vi "FPGA.vi"(7 "LabVIEW Web Service Request":refnum<class "Web Request.lvclass">, 9 "getdata":dbl, 10 "stop":dbl, 11 "save_file":dbl) -> (1 "Chassis Temperature":dbl, 2 "value":string)   [LabVIEW 2020]
uses:
  <vilib>/wsapi/Web Request.lvclass
panel:
  # "Use the Web Service Request input terminal to call the VIs on the Web Services palette. Do not remove it from the connector pane unless you don't need access to the palette."
  # "Each additional control wired to the connector pane will be available as an input in the URL. To include an indicator in terminal-mode output (the default setting), it must also be wired to the connector pane."
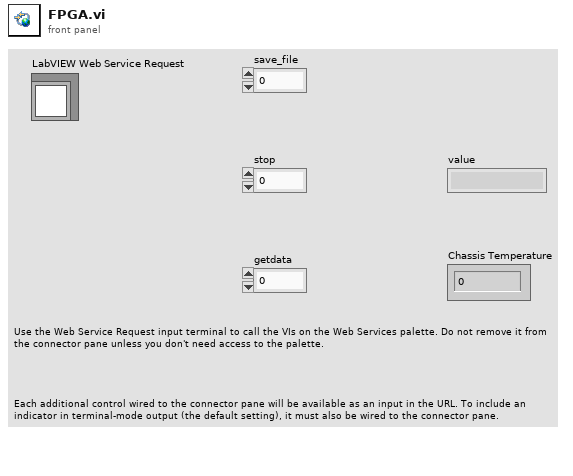
[diagram p1: front panel]
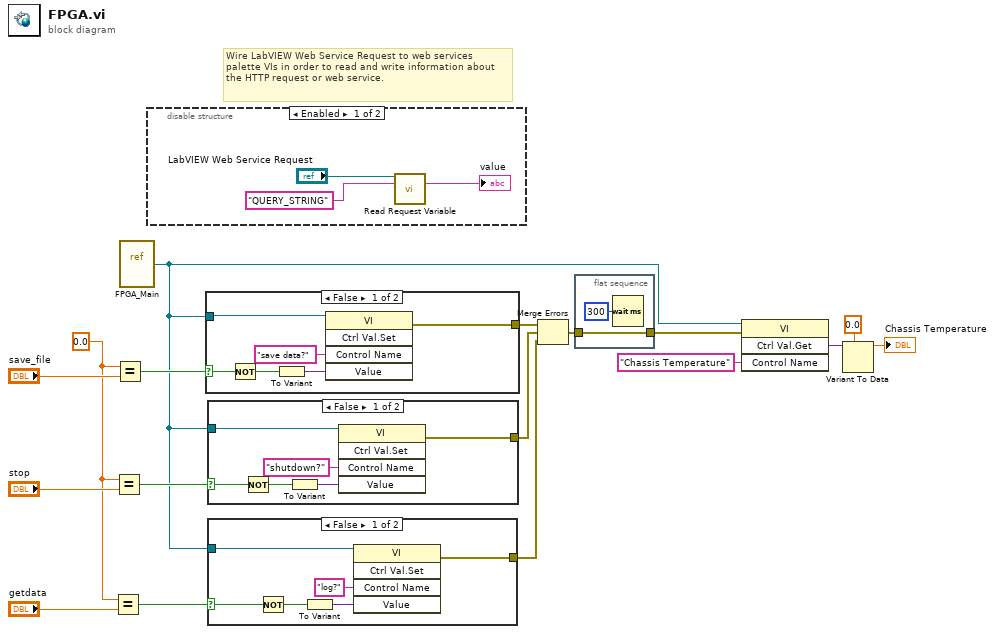
[diagram p0: block diagram]
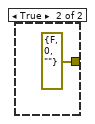
[diagram p2: hidden frame]
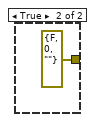
[diagram p3: hidden frame]
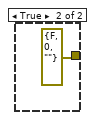
[diagram p4: hidden frame]
diagram:
  w10 = 0.0 ("x")
  # "Wire LabVIEW Web Service Request to web services palette VIs in order to read and write information about the HTTP request or web service."
  n1 = Equal?(x=w10, y="getdata") -> (x = y?=w8:bool)
  n2 = Equal?(x=w10, y="stop") -> (x = y?=w7:bool)
  n3 = Equal?(x=w10, y="save_file") -> (x = y?=w9:bool)
  n4 = vi-ref "FPGA_Main.vi"() -> (w6:refnum<vi>)
  n5 = disable-structure shown="Enabled" {
    frame Enabled {
      n6 = call <vilib>:"Read Request Variable.vi"("LabVIEW Web Service Request"="LabVIEW Web Service Request", "variable name"="QUERY_STRING") -> ("value"=→"value":string)  [unwired: 11 in, 2 out]
    }
    frame Disabled {
    }
  }
  n7 = case shown="False" w9 {
    selector: w9 -> [w25 _]
    tunnel: w6 -> [w26 _]
    tunnel: [w21 errorcluster {"status"=FALSE, "code"=0, "source"=""} ("error out")] -> w3
    frame False {
      n8 = Not(x=w25) -> (.not. x?=w23:bool)
      n9 = To Variant(anything=w23) -> (Variant=w24:variant)
      n10 = invoke class="VI" method="Ctrl Val.Set"(reference=w26, "Control Name"="save data?", "Value"=w24) -> (error out=w21:errorcluster)  [unwired: 2 in, 4 out]
    }
    frame True {
    }
  }
  n11 = case shown="False" w7 {
    selector: w7 -> [w30 _]
    tunnel: w6 -> [w29 _]
    tunnel: [w28 errorcluster {"status"=FALSE, "code"=0, "source"=""} ("error out")] -> w4
    frame False {
      n12 = Not(x=w30) -> (.not. x?=w32:bool)
      n13 = To Variant(anything=w32) -> (Variant=w31:variant)
      n14 = invoke class="VI" method="Ctrl Val.Set"(reference=w29, "Control Name"="shutdown?", "Value"=w31) -> (error out=w28:errorcluster)  [unwired: 2 in, 4 out]
    }
    frame True {
    }
  }
  n15 = case shown="False" w8 {
    selector: w8 -> [w37 _]
    tunnel: w6 -> [w36 _]
    tunnel: [w35 errorcluster {"status"=FALSE, "code"=0, "source"=""} ("error out")] -> w5
    frame False {
      n16 = Not(x=w37) -> (.not. x?=w39:bool)
      n17 = To Variant(anything=w39) -> (Variant=w40:variant)
      n18 = invoke class="VI" method="Ctrl Val.Set"(reference=w36, "Control Name"="log?", "Value"=w40) -> (error out=w35:errorcluster)  [unwired: 2 in, 4 out]
    }
    frame True {
    }
  }
  n19 = Merge Errors(w3, w4, w5) -> (w2:errorcluster)
  n20 = flat-sequence {
    tunnel: w2 -> [w42]
    tunnel: [w42] -> w1
    frame #0 {
      n21 = Wait (ms)(milliseconds to wait=u32 300) -> ()  [unwired: 1 out]
    }
  }
  n22 = invoke class="VI" method="Ctrl Val.Get"(reference=w6, error in=w1, "Control Name"="Chassis Temperature") -> ("Get Control Value Variant"=w16:variant)  [unwired: 1 in, 3 out]
  n23 = Variant To Data(type=0.0, Variant=w16) -> (data=→"Chassis Temperature":dbl)  [unwired: 1 in, 1 out]
